vi "handle_error.vi"(8 "error in (no error)":errorcluster, 11 "scan_panel in":refnum<class "scan_panel.lvclass">) -> (0 "error out":errorcluster, 3 "scan_panel out":refnum<class "scan_panel.lvclass">)   [LabVIEW 2015, in "scan_panel.lvclass"]
uses:
  scan_panel.lvclass
  scan_panel.lvclass/scan_panel.ctl
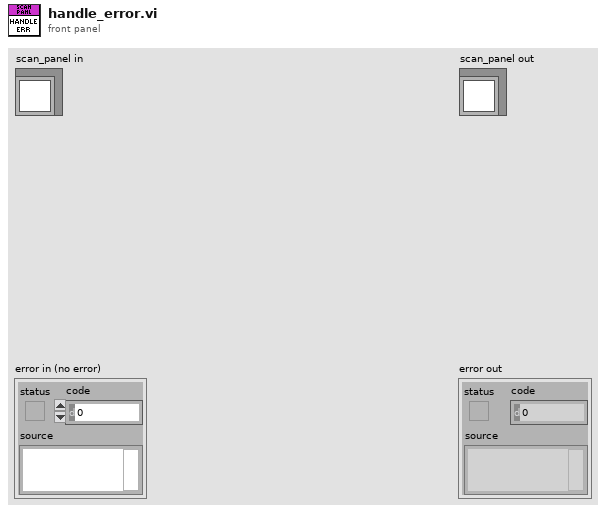
[diagram p1: front panel]
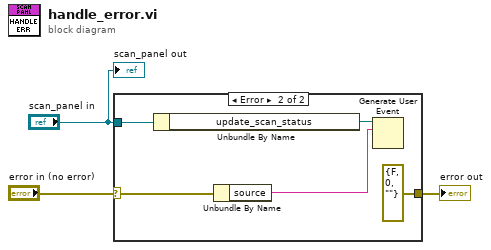
[diagram p0: block diagram]
diagram:
  n1 = case shown="Error" "error in (no error)" {
    selector: "error in (no error)" -> [w4 w6]
    tunnel: "scan_panel in" -> [_ w9]
    tunnel: [w4 errorcluster {"status"=FALSE, "code"=0, "source"=""} ("error IO")] -> w1
    frame No Error {
    }
    frame Error {
      n2 = Unbundle By Name(w9) -> ("update_scan_status"=w8:refnum<user-event>)
      n3 = Unbundle By Name(w6) -> ("source"=w7:string)
      n4 = Generate User Event(user event=w8, event data cluster=w7) -> ()  [unwired: 2 in, 2 out]
    }
  }
  "error out" <- w1
  "scan_panel out" <- "scan_panel in"
